vi "Cool Down Start.vi"() -> ()   [LabVIEW 2014]
panel:
  out "?":string="Close Me After LabView Starts"
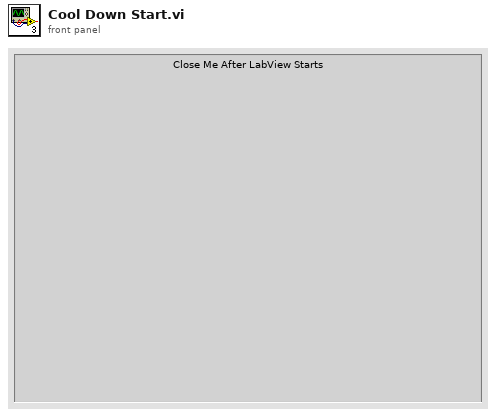
[diagram p1: front panel]
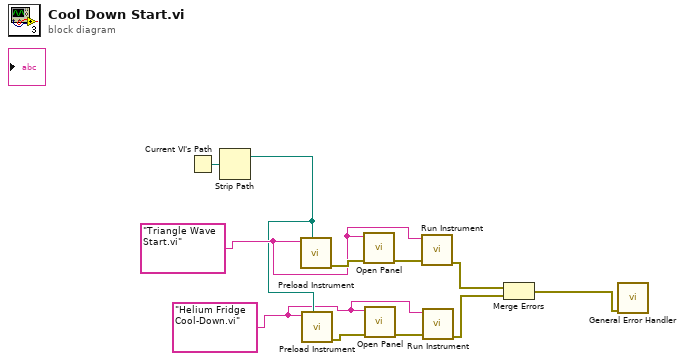
[diagram p0: block diagram]
diagram:
  w4 = "Helium Fridge Cool-Down.vi"
  w9 = "Triangle Wave Start.vi"
  n1 = Current VI's Path() -> (path=w11:path)
  n2 = Strip Path(path=w11) -> (stripped path=w5:path)  [unwired: 1 out]
  n3 = call <vilib>:"Preload Instrument.vi"("VI path"=w5, "VI name"=w9) -> ("error out"=w10:errorcluster)  [unwired: 9 in]
  n4 = call <vilib>:"Preload Instrument.vi"("VI path"=w5, "VI name"=w4) -> ("error out"=w7:errorcluster)  [unwired: 9 in]
  n5 = call <vilib>:"Open Panel.vi"("error in (no error)"=w10, "VI name"=w9) -> ("error out"=w8:errorcluster)  [unwired: 9 in]
  n6 = call <vilib>:"Open Panel.vi"("error in (no error)"=w7, "VI name"=w4) -> ("error out"=w6:errorcluster)  [unwired: 9 in]
  n7 = call <vilib>:"Run Instrument.vi"("error in (no error)"=w8, "VI name"=w9) -> ("error out"=w3:errorcluster)  [unwired: 9 in]
  n8 = call <vilib>:"Run Instrument.vi"("error in (no error)"=w6, "VI name"=w4) -> ("error out"=w2:errorcluster)  [unwired: 9 in]
  n9 = Merge Errors(w3, w2) -> (w1:errorcluster)
  n10 = call <vilib>:"General Error Handler.vi"("error in (no error)"=w1) -> ()  [unwired: 10 in, 5 out]
